vi "PID Autotuning (Temperature).vi"(0 "desired temperature":dbl format="%.2f", 1 "measured temperature":dbl format="%.2f", 2 "plant parameters in":T1={"process gain"=1.0, "time constant (s)"=0.01, "delay time (s)"=0.0} {"delay time (s)" format="%.3f"; "time constant (s)" format="%.3f"; "process gain" format="%.3f"}, 3 "autotune? (F)":bool, 4 "PID gains in":T2={"proportional gain (Kc)"=1.0, "integral time (Ti, min)"=0.01, "derivative time (Td, min)"=0.0} {"derivative time (Td, min)" format="%.3f"; "integral time (Ti, min)" format="%.3f"; "proportional gain (Kc)" format="%.3f"}, 5 "dt (s)":dbl=-1.0 format="%.3f", 6 "output range":cluster{"output high":dbl, "output low":dbl}={"output high"=100.0, "output low"=-100.0} {"output low" format="%.2f"; "output high" format="%.2f"}, 7 "reinitialize? (F)":bool, 8 "auto? (T)":bool=TRUE, 9 "beta":dbl=1.0 format="%.2f", 10 "manual control":dbl format="%.2f", 11 "autotuning parameters":T3={"type of controller"=0, "time constant factor"=2.0, "step amplitude"=1.0} {"step amplitude" format="%.2f"; "type of controller" items=["P", "PI", "PID"]}, 13 "alpha":dbl=0.1 format="%.2f") -> (14 "output":dbl format="%.2f", 15 "tuning completed?":bool, 16 "plant parameters out":T1={"process gain"=1.0, "time constant (s)"=0.01, "delay time (s)"=0.0} {"delay time (s)" format="%.3f"; "time constant (s)" format="%.3f"; "process gain" format="%.3f"}, 18 "PID gains out":T2={"proportional gain (Kc)"=1.0, "integral time (Ti, min)"=0.01, "derivative time (Td, min)"=0.0} {"derivative time (Td, min)" format="%.3f"; "integral time (Ti, min)" format="%.3f"; "proportional gain (Kc)" format="%.3f"})   [LabVIEW 2017, in "NI_PID_autopid.lvlib"]
doc: "Directly controls and tunes a system. You can use this VI to improve performance of not only temperature systems, but also other types of systems that contain dead time. This VI uses internal model control to compensate for dead time and tune the system."
uses:
  <vilib>/addons/control/pid/NI_PID_autopid.lvlib
  <vilib>/addons/control/pid/autopid.llb/PID autotuning parameters (FO).ctl
  <vilib>/addons/control/pid/pid.llb/PID Structure Conversion (DBL).vi
  <vilib>/addons/control/pid/pid.llb/PID Lead-Lag (DBL).vi
  <vilib>/addons/control/pid/pid.llb/PID Advanced (DBL).vi
  <vilib>/addons/control/pid/NI_PID_pid.lvlib
  <vilib>/addons/control/advanced/NI_AdvCtrl_nonlinear.lvlib
  <vilib>/ptbypt/NI_PtbyPt.lvlib
panel:
  out "dt out (s)":dbl format="%.3f"
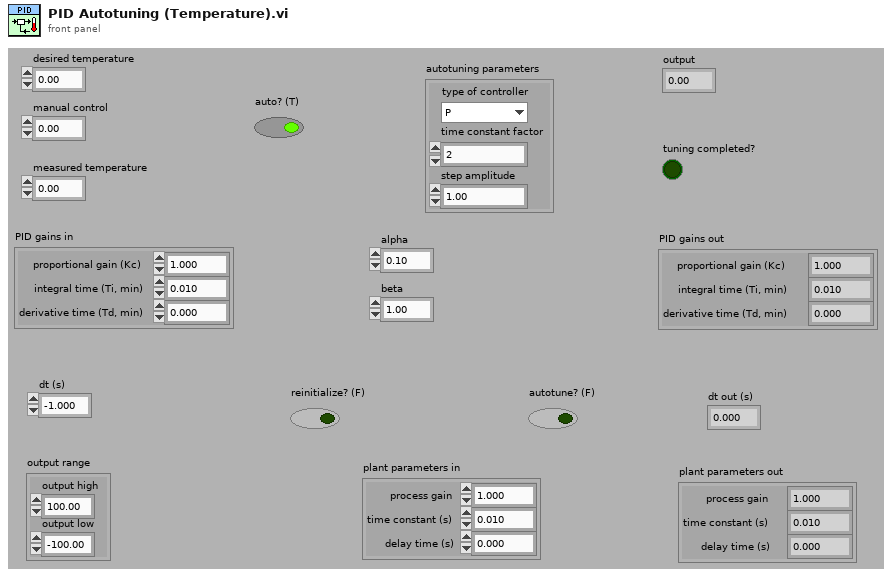
[diagram p1: front panel]
types:
  T1 = cluster{"process gain":dbl, "time constant (s)":dbl, "delay time (s)":dbl}
  T2 = cluster{"proportional gain (Kc)":dbl, "integral time (Ti, min)":dbl, "derivative time (Td, min)":dbl}
  T3 = typedef "NI_PID_autopid.lvlib/PID autotuning parameters (FO).ctl" = cluster{"type of controller":u16, "time constant factor":dbl, "step amplitude":dbl}
  T4 = cluster{"Plant Gain (K)":dbl, "Time Constant (T)":dbl, "Dead Time (L)":dbl}
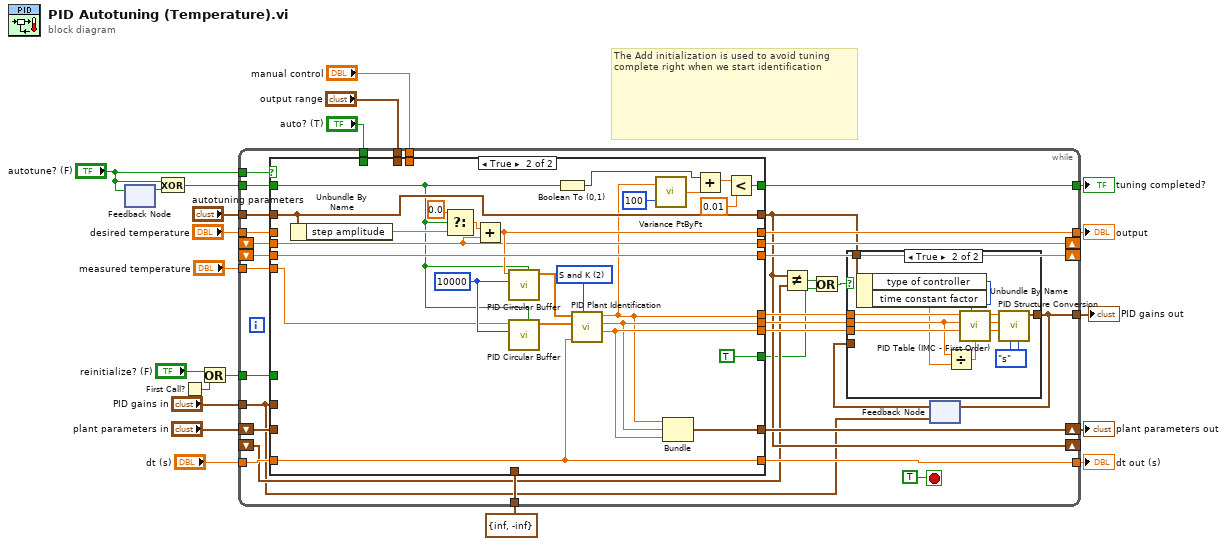
[diagram p0: block diagram]
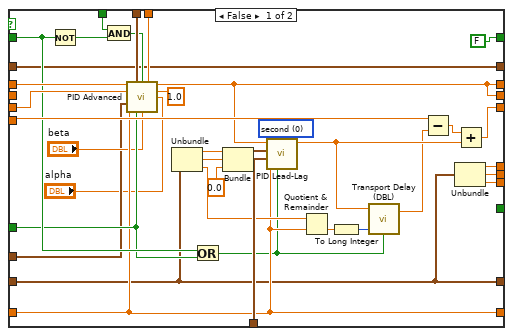
[diagram p3: hidden frame]
diagram:
  # "The Add initialization is used to avoid tuning complete right when we start identification"
  n1 = feedback #1() -> (w8:bool)  [unwired: 1 in]
  n2 = feedback-in #1("autotune? (F)") -> ()
  n3 = Exclusive Or(1:w8, 2:"autotune? (F)") -> (0:w6:bool)
  n4 = First Call?() -> (First Call?: T/F=w14:bool)
  n5 = Or(x="reinitialize? (F)", y=w14) -> (x .or. y?=w12:bool)
  n6 = while {
    tunnel: "desired temperature" -> [w46]
    tunnel: "measured temperature" -> [w50]
    tunnel: "output range" -> [w48]
    tunnel: "dt (s)" -> [w44]
    tunnel: w12 -> [w43]
    tunnel: "autotune? (F)" -> [w37]
    tunnel: [w34] -> w17
    tunnel: [w25] -> w16
    shift-right: [w51] -> _
    shift-left: _ -> [w49]
    tunnel: cluster{"output high":dbl, "output low":dbl} {"output high"=inf, "output low"=-inf} ("output range 2") -> [w47]
    shift-right: [w52] -> _
    shift-left: _ -> [w38]
    tunnel: "autotuning parameters" -> [w40]
    tunnel: "auto? (T)" -> [w42]
    tunnel: "manual control" -> [w41]
    tunnel: w6 -> [w39]
    shift-right: [w36] -> w4
    shift-left: "plant parameters in" -> [w45]
    tunnel: [w35] -> w5
    shift-right: [w29] -> _
    shift-left: _ -> [w28]
    tunnel: "PID gains in" -> [w23]
    tunnel: [w22] -> w1
    stop <- TRUE stop-if-true
    n7 = case shown="True" w37 {
      tunnel: [w83 w120] -> w52
      tunnel: [w93 w123] -> w51
      tunnel: w50 -> [w95 w105]
      tunnel: w49 -> [w92 w123]
      tunnel: w48 -> [w102 _]
      tunnel: w47 -> [w101 _]
      tunnel: w46 -> [w100 _]
      tunnel: w45 -> [w81 _]
      tunnel: w44 -> [w85 w116]
      tunnel: w43 -> [w90 _]
      tunnel: w42 -> [w97 _]
      tunnel: w41 -> [w99 _]
      tunnel: w40 -> [w82 w112]
      tunnel: w39 -> [w91 w107]
      tunnel: w38 -> [_ w120]
      tunnel: [w81 w122] -> w36
      tunnel: [w83 w121] -> w35
      tunnel: [w85 w116] -> w34
      tunnel: [FALSE ("tuning status") w109] -> w25
      tunnel: [w82 w112] -> w29
      tunnel: [w80 w104] -> w33
      tunnel: [w79 w114] -> w31
      tunnel: [w78 w115] -> w32
      tunnel: [_ TRUE ("y")] -> w26
      tunnel: w23 -> [w73 _]
      frame False {
        w72 = u16 0 items=["second", "minute"] ("time unit")
        n8 = Not(x=w91) -> (.not. x?=w67:bool)
        n9 = And(x=w97, y=w67) -> (x .and. y?=w96:bool)
        n10 = call-poly <vilib>:"PID Advanced.vi"("setpoint"=w100, "output range"=w102, "auto? (T)"=w96, "manual control"=w99, "process variable"=w92, "gamma"=1.0 ("Gamma"), "alpha"="alpha", "PID gains"=w73, "dt (s)"=w85, "reinitialize? (F)"=w90, "beta"="beta") -> ("output"=w83:dbl)  [unwired: 3 in, 1 out]
        n11 = Unbundle(w81) -> ("Plant Gain (K)"=w89:dbl, "Time Constant (T)"=w71:dbl, "Dead Time (L)"=w86:dbl)
        n12 = Or(x=w91, y=w90) -> (x .or. y?=w70:bool)
        n13 = Bundle("Plant Gain (K)"=w89, "Time Constant (T)"=w71, "Dead Time (L)"=0.0) -> (w87:T4)  [unwired: 1 in]
        n14 = call-poly <vilib>:"PID Lead-Lag.vi"("reinitialize? (F)"=w70, "time unit"=w72, "dt (s)"=w85, "output range"=w101, "tuning parameters"=w87, "input"=w83) -> ("output"=w77:dbl)  [unwired: 2 in, 1 out]
        n15 = Quotient & Remainder(x=w86, y=w85) -> (floor(x/y)=w98:dbl)  [unwired: 1 out]
        n16 = To Long Integer(number=w98) -> (32bit integer=w68:i32)
        n17 = call <vilib>:"Transport Delay (DBL).vi"("initialize"=w70, "delay"=w68, "input point"=w77) -> ("output point"=w76:dbl)  [unwired: 2 in]
        n18 = Subtract(x=w95, y=w76) -> (x-y=w94:dbl)
        n19 = Unbundle(w81) -> ("Plant Gain (K)"=w80:dbl, "Time Constant (T)"=w79:dbl, "Dead Time (L)"=w78:dbl)
        n20 = Add(x=w94, y=w77) -> (x+y=w93:dbl)
      }
      frame True {
        w124 = 10000 ("sample length")
        w119 = u16 2 items=["Z-N", "First Order", "S and K"] ("Ring")
        n21 = Unbundle By Name(w112) -> ("step amplitude"=w126:dbl)
        n22 = Select(t=0.0, s=w107, f=w126) -> (s? t:f=w125:dbl)
        n23 = Add(x=w125, y=w120) -> (x+y=w121:dbl)
        n24 = call <vilib>:"PID Circular Buffer.vi"("initialize"=w107, "sample length"=w124, "input data point"=w121) -> ("Current Queue"=w118:dbl[])  [unwired: 7 in, 1 out]
        n25 = call <vilib>:"PID Circular Buffer.vi"("initialize"=w107, "sample length"=w124, "input data point"=w105) -> ("Current Queue"=w117:dbl[])  [unwired: 7 in, 1 out]
        n26 = Boolean To (0,1)(Boolean=w107) -> (0, 1=w106:i16)
        n27 = call <vilib>:"PID Plant Identification.vi"("Method"=w119, "Sampling Time"=w116, "Response signal"=w117, "Stimulus signal"=w118) -> ("Dead Time (L)"=w115:dbl, "Time Constant (T)"=w114:dbl, "Plant Gain (K)"=w104:dbl)  [unwired: 1 in, 4 out]
        n28 = call <vilib>:"Variance PtByPt.vi"("x"=w104, "sample length"=100) -> ("variance"=w111:dbl)  [unwired: 1 in, 2 out]
        n29 = Bundle("Plant Gain (K)"=w104, "Time Constant (T)"=w114, "Dead Time (L)"=w115) -> (w122:T4)  [unwired: 1 in]
        n30 = Add(x=w106, y=w111) -> (x+y=w108:dbl)
        n31 = Less?(x=w108, y=0.01) -> (x < y?=w109:bool)
      }
    }
    n32 = Not Equal?(x=w29, y=w28) -> (x != y?=w30:bool)
    n33 = Or(x=w30, y=w26) -> (x .or. y?=w27:bool)
    n34 = feedback #2(w23) -> (w24:T2)
    n35 = case shown="True" w27 {
      tunnel: [w54 w60] -> w22
      tunnel: w33 -> [_ w59]
      tunnel: w32 -> [_ w58]
      tunnel: w31 -> [_ w57]
      tunnel: w29 -> [_ w56]
      tunnel: w24 -> [w54 _]
      frame False {
      }
      frame True {
        w65 = enum16{"min", "s"}."s" ("integral unit")
        n36 = Unbundle By Name(w56) -> ("type of controller"=w61:u16, "time constant factor"=w55:dbl)
        n37 = Divide(x=w57, y=w55) -> (x/y=w66:dbl)
        n38 = call <vilib>:"PID Table (IMC - First Order).vi"("Desired Time Constant (tau_c)"=w66, "Type of Controller"=w61, "Plant delay (theta)"=w58, "Plant time constant (tau)"=w57, "Plant gain (K)"=w59) -> ("TD"=w64:dbl, "Ti"=w63:dbl, "Kc"=w62:dbl)  [unwired: 4 in]
        n39 = call-poly <vilib>:"PID Structure Conversion.vi"("derivative unit"=w65, "integral unit"=w65, "derivative"=w64, "integral"=w63, "proportional"=w62) -> ("PID gains"=w60:T2)  [unwired: 6 in]
      }
    }
    n40 = feedback-in #2(w22) -> ()
  }
  "output" <- w5
  "dt out (s)" <- w17
  "PID gains out" <- w1
  "tuning completed?" <- w16
  "plant parameters out" <- w4
